vi "Set Harmonic.vi"(8 "error in (no error)":errorcluster, 9 "Fundamental (T: Primary (Normal))":bool=TRUE, 10 "Harmonic Value (1)":i32=1, 11 "VISA resource name":refnum<visa-resource-name>) -> (0 "error out":errorcluster, 3 "VISA resource name out":refnum<visa-resource-name>)   [LabVIEW 2011, in "Fluke 5XXX Series Multicalibrators.lvlib"]
doc: "This VI makes the frequency of one output a multiple of another output for the ac voltage or ac power functions (sinewaves only).\n\nFor example, in dual ac voltage, have the frequency of the voltage output on the Calibrator front panel NORMAL terminals at 60 Hz and the frequency of the voltage output on the AUX terminals at the 7th harmonic (420 Hz). The range for the harmonics is 1 to 50.\n\nNote:\n\nThis VI is available only for instrument models 5500A and 5520A."
uses:
  Fluke 5XXX Series Multicalibrators.lvlib
panel:
  # "Primary (Normal)"
  # "Secondary (Auxiliary)"
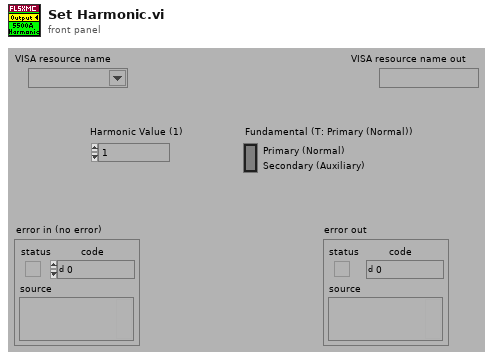
[diagram p1: front panel]
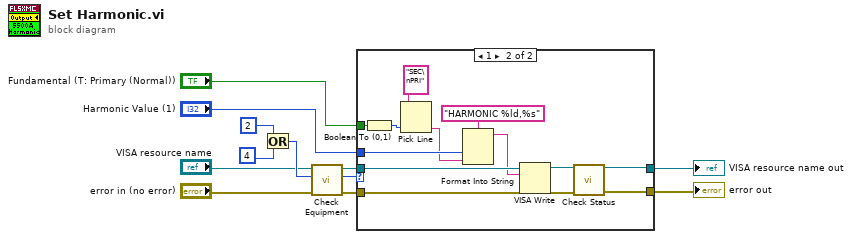
[diagram p0: block diagram]
diagram:
  n1 = Or(x=2 ("Numeric"), y=4 ("Numeric")) -> (x .or. y?=w9:i32)
  n2 = call "Check Equipment.vi"("error in (no error)"="error in (no error)", "Bit Mask"=w9, "VISA resource name"="VISA resource name") -> ("error out"=w12:errorcluster, "Present?"=w11:u32, "VISA resource name out"=w10:refnum<visa-resource-name>)  [unwired: 6 in]
  n3 = case shown="1" w11 {
    tunnel: [w13 w22] -> w5
    tunnel: w12 -> [w14 w27]
    tunnel: w10 -> [w13 w26]
    tunnel: [w14 w25] -> w6
    tunnel: "Fundamental (T: Primary (Normal))" -> [_ w19]
    tunnel: "Harmonic Value (1)" -> [_ w18]
    frame 0, Default {
    }
    frame 1 {
      n4 = Boolean To (0,1)(Boolean=w19) -> (0, 1=w16:i16)
      n5 = Pick Line(multi-line string="SEC\nPRI", line index=w16) -> (output string=w17:string)  [unwired: 1 in]
      n6 = Format Into String(format string="HARMONIC %ld,%s", w18, w17) -> (resulting string=w20:string)  [unwired: 2 in, 1 out]
      n7 = VISA Write(VISA resource name=w26, write buffer=w20, error in (no error)=w27) -> (VISA resource name out=w23:refnum<visa-resource-name>, error out=w24:errorcluster)  [unwired: 1 out]
      n8 = call "Check Status.vi"("VISA resource name"=w23, "error in (no error)"=w24) -> ("VISA resource name out"=w22:refnum<visa-resource-name>, "error out"=w25:errorcluster)  [unwired: 12 in]
    }
  }
  "VISA resource name out" <- w5
  "error out" <- w6
